vi "Reference Method Dialog.vi"(8 "Start Path":path) -> (0 "Path out":path, 1 "Cancelled?":bool, 3 "Use Reference Method out":bool)   [LabVIEW 2020, in "Message Rescripter.lvlib"]
uses:
  Message Rescripter.lvlib
  Localized Strings.vi
panel:
  out "Path Display":string
  in  "Path":path caption="Select a path to the reference method."
  in  "Use Reference Method":bool
  in  "Cancel Button":bool
  in  "OK Button":bool
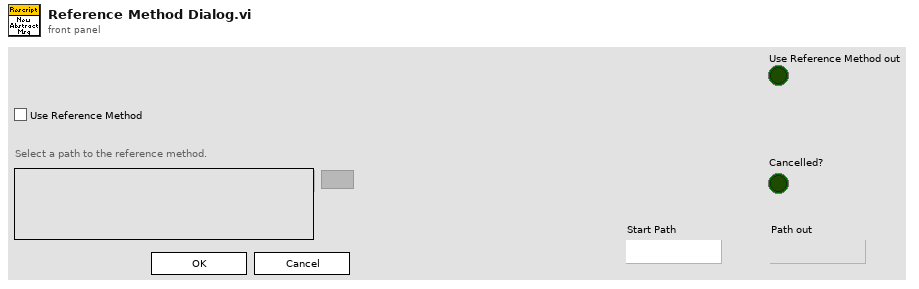
[diagram p1: front panel]
types:
  T1 = enum8{"Enabled", "Disabled", "Disabled and Grayed Out"}
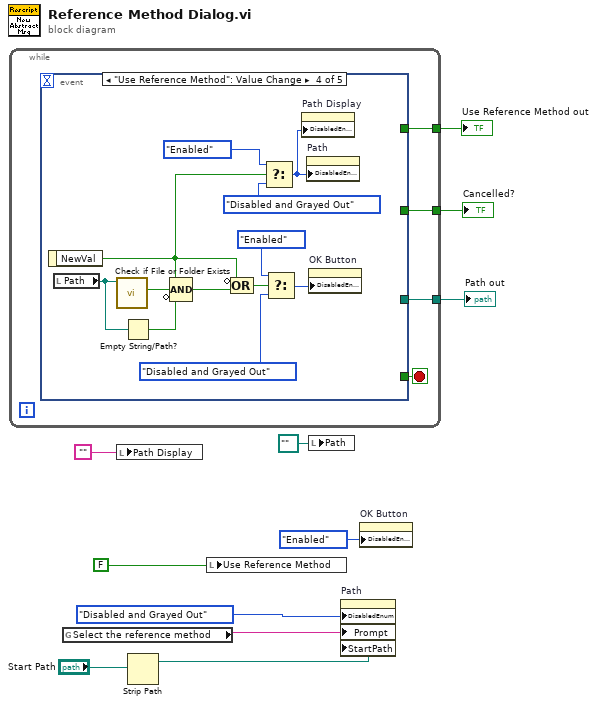
[diagram p0: block diagram]
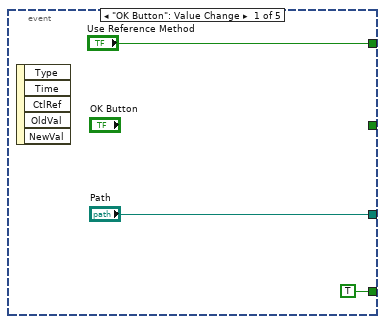
[diagram p2: hidden frame]
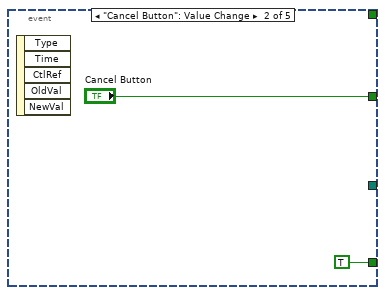
[diagram p3: hidden frame]
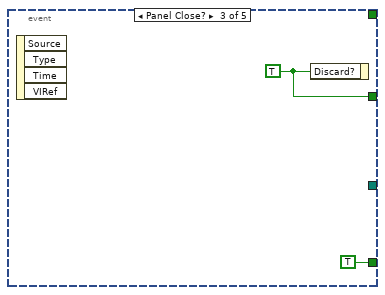
[diagram p4: hidden frame]
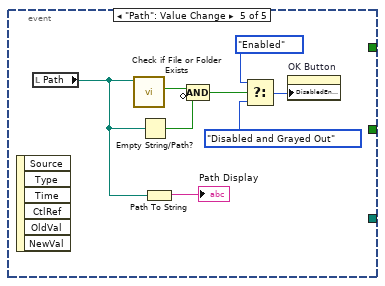
[diagram p5: hidden frame]
diagram:
  n1 = while {
    tunnel: [w15] -> w11
    tunnel: [w14] -> w10
    tunnel: [w13] -> w8
    stop <- w12 stop-if-true
    n2 = event shown="[3] \"Use Reference Method\": Value Change" {
      selector: _ -> [_ _ _ _ _]
      dyn-events: _ -> [_ _ _ _ _]
      timeout: _ -> [_ _ _ _ _]
      tunnel: [_ "Cancel Button" w22 _ _] -> w15
      tunnel: ["Use Reference Method" _ _ _ _] -> w14
      tunnel: ["Path" _ _ _ _] -> w13
      tunnel: [TRUE TRUE TRUE _ _] -> w12
      event "OK Button": Value Change {
        n3 = event-data() -> ()  [unwired: 1 in, 5 out]
      }
      event "Cancel Button": Value Change {
        n4 = event-data() -> ()  [unwired: 1 in, 5 out]
      }
      event Panel Close? {
        w22 = TRUE ("Discard?")
        n5 = event-data() -> ()  [unwired: 1 in, 4 out]
        n6 = event-data("Discard?"=w22) -> ()  [unwired: 1 in, 1 out]
      }
      event "Use Reference Method": Value Change {
        n7 = event-data() -> ("NewVal"=w24:bool)  [unwired: 1 in]
        n8 = local read "Path"() -> (w26:path)
        n9 = call <vilib>:"Check if File or Folder Exists.vi"("path"=w26) -> ("file or folder exists?"=w27:bool)  [unwired: 8 in, 2 out]
        n10 = Empty String/Path?(string/path=w26) -> (empty?=w25:bool)
        n11 = Compound Arithmetic op=AND(w24, w27, invert w25) -> (w29:bool)
        n12 = Compound Arithmetic op=OR(invert w24, w29) -> (w28:bool)
        n13 = Select(t=T1."Enabled", s=w24, f=T1."Disabled and Grayed Out" ("Disabled")) -> (s? t:f=w23:T1)
        n14 = Select(t=T1."Enabled", s=w28, f=T1."Disabled and Grayed Out" ("Disabled")) -> (s? t:f=w32:T1)
        n15 = property on="Path Display" class="Str"("DisabledEnum"=w23) -> ()  [unwired: 2 in, 2 out]
        n16 = property on="Path" class="Path"("DisabledEnum"=w23) -> ()  [unwired: 2 in, 2 out]
        n17 = property on="OK Button" class="Bool"("DisabledEnum"=w32) -> ()  [unwired: 2 in, 2 out]
      }
      event "Path": Value Change {
        n18 = event-data() -> ()  [unwired: 1 in, 6 out]
        n19 = local read "Path"() -> (w35:path)
        n20 = call <vilib>:"Check if File or Folder Exists.vi"("path"=w35) -> ("file or folder exists?"=w39:bool)  [unwired: 8 in, 2 out]
        n21 = Empty String/Path?(string/path=w35) -> (empty?=w38:bool)
        n22 = Path To String(path=w35) -> (string=→"Path Display":string)
        n23 = Compound Arithmetic op=AND(w39, invert w38) -> (w37:bool)
        n24 = Select(t=T1."Enabled", s=w37, f=T1."Disabled and Grayed Out" ("Disabled")) -> (s? t:f=w42:T1)
        n25 = property on="OK Button" class="Bool"("DisabledEnum"=w42) -> ()  [unwired: 2 in, 2 out]
      }
    }
  }
  "Cancelled?" <- w11
  "Use Reference Method out" <- w10
  "Path out" <- w8
  n26 = global read "Localized Strings.vi" "Select the reference method"() -> (w1:string)
  n27 = local write "Path Display"("" ("Name")) -> ()
  n28 = Strip Path(path="Start Path") -> (stripped path=w5:path)  [unwired: 1 out]
  n29 = local write "Use Reference Method"(FALSE ("Use Reference Method")) -> ()
  n30 = local write "Path"(path "" ("Path")) -> ()
  n31 = property on="Path" class="Path"("DisabledEnum"=T1."Disabled and Grayed Out" ("Disabled"), "Prompt"=w1, "StartPath"=w5) -> ()  [unwired: 2 in, 2 out]
  n32 = property on="OK Button" class="Bool"("DisabledEnum"=T1."Enabled" ("Disabled")) -> ()  [unwired: 2 in, 2 out]
